vi "CSM - Request CSM to Post Message.vi"(4 "Immediately?(F)":bool, 6 "Without Reply?(F)":bool, 7 "Module Name":string, 8 "Error In (no error)":errorcluster, 9 "Target Module(\"\" by Default)":string, 10 "Arguments (\"\")":string, 11 "State":string) -> (0 "error out":errorcluster)   [LabVIEW 2020, in "Communicable State Machine.lvlib"]
doc: "Request CSM to Post a message to CSM specified. This is usually used in sub-loops with a CSM for acting as a holistic module.\n\n<b>Inputs:</b>\n - <b>Status</b>: Message to post.\n - <b>Arguments (\"\")</b>: Argument of the message.\n - <b>Target Module</b>:Target CSM module name.\n - <b>Module Name</b>:Host Module Name\n - <b>Error In (no error)</b>: Error cluster\n\n<b>Outputs:</b>\n - <b>error out</b>: Error cluster"
uses:
  Communicable State Machine.lvlib
  _CSM_MSG_TYPE.ctl
  CSM - Message Type.ctl
  _Cross CSM State Data.ctl
  _Cross CSM State Response.ctl
  _CSM_Response Source Message.ctl
  _CSMOFGVOPER.ctl
  Priority Queue.lvclass/Priority Queue.ctl
  Priority Queue.lvclass
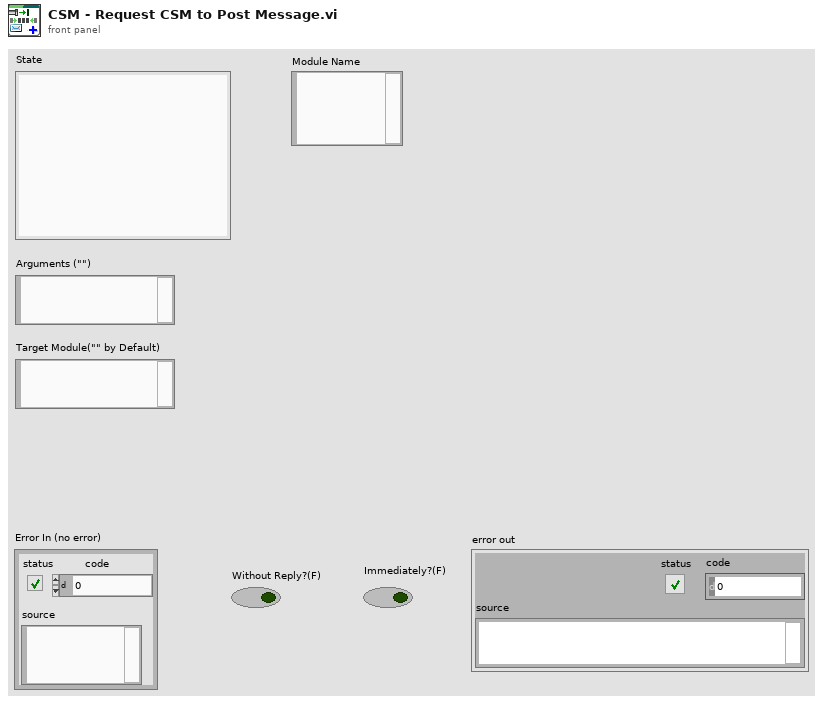
[diagram p1: front panel]
types:
  T1 = typedef "Communicable State Machine.lvlib/_CSM_MSG_TYPE.ctl" = enum16{"Sync Message(-@)", "Async Message(->)", "Async without Response(->|)", "Async Response", "Broadcast(-><all>)", "Broadcast(-><status>)", "Broadcast(-><interrupt>)", "Append to JKISM States", "Append to JKISM States(High Priority)"}
  T2 = typedef "Communicable State Machine.lvlib/CSM - Message Type.ctl" = enum16{"Async", "Async without Reply", "Sync"}
  T3 = typedef "Communicable State Machine.lvlib/_Cross CSM State Data.ctl" = cluster{"Msg Type":T1, "state":string, "args":string, "source":string, "RespQ":refnum<queue>, "Response For Message":T4, "Target":string}
  T4 = typedef "Communicable State Machine.lvlib/_CSM_Response Source Message.ctl" = cluster{"‘State":string, "’Arguments":string, "’Error":errorcluster}
  T5 = typedef "Communicable State Machine.lvlib/_CSMOFGVOPER.ctl" = enum16{"Create If not Exist", "Get By Name", "List", "Check If Name Exists", "Release", "Module Status", "Create Status Event Handler", "Destroy Status Event Handler"}
  T6 = typedef "Communicable State Machine.lvlib/_CSMObj.ctl" = cluster{"Requested Name":string, "Module Name":string, "Mode":T7, "Queue":refnum<class "Priority Queue.lvclass">, "CSM-Data":refnum<data-value>, "User Event":refnum<user-event>, "Status Change Event":refnum<user-event>, "Allowed Messages":string[], "Mode-Data":refnum<data-value>, "Group Name":string, "Exit Event":refnum<user-event>}
  T7 = typedef "Communicable State Machine.lvlib/_CSM_MODE.ctl" = enum16{"Not Exist", "Stand Alone", "CSM", "Worker Agent", "Worker", "Chain", "Chain Node"}
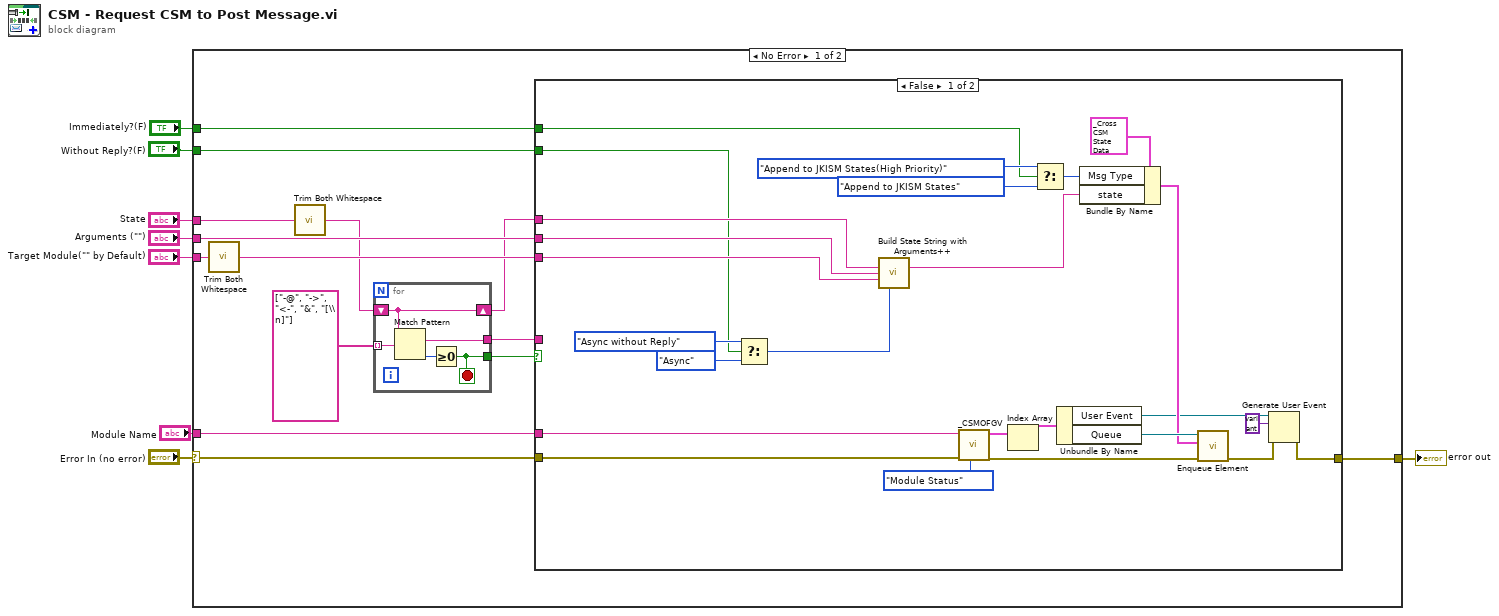
[diagram p0: block diagram]
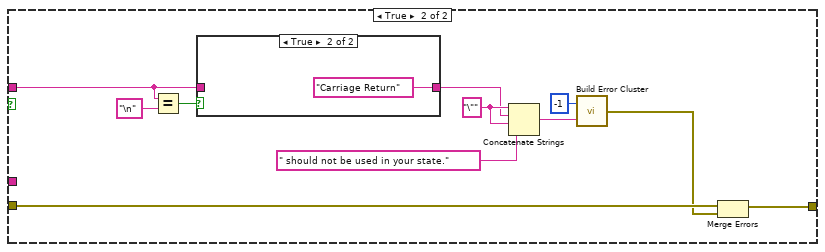
[diagram p2: hidden frame]
diagram:
  n1 = case shown="No Error" "Error In (no error)" {
    selector: "Error In (no error)" -> [w20 w66]
    tunnel: "State" -> [w17 _]
    tunnel: [w21 w66] -> w6
    tunnel: "Arguments (\"\")" -> [w18 _]
    tunnel: "Target Module(\"\" by Default)" -> [w22 _]
    tunnel: "Module Name" -> [w16 _]
    tunnel: "Without Reply?(F)" -> [w15 _]
    tunnel: "Immediately?(F)" -> [w9 _]
    frame No Error {
      n2 = call "Trim Both Whitespace.vi"("string"=w22) -> ("trimmed string"=w19:string)  [unwired: 1 in]
      n3 = call "Trim Both Whitespace.vi"("string"=w17) -> ("trimmed string"=w10:string)  [unwired: 1 in]
      n4 = for {
        shift-right: [w65] -> w13
        shift-left: w10 -> [w65]
        tunnel: string[] ["-@", "->", "<-", "&", "[\\n]"] -> [w64] mode=indexing
        tunnel: [w62] -> w11
        tunnel: [w61] -> w12
        stop <- w61 stop-if-true
        n5 = Match Pattern(string=w65, regular expression=w64) -> (match substring=w62:string, offset past match=w63:i32)  [unwired: 1 in, 2 out]
        n6 = Greater Or Equal To 0?(x=w63) -> (x >= 0?=w61:bool)
      }
      n7 = case shown="False" w12 {
        tunnel: w18 -> [w32 _]
        tunnel: w19 -> [w31 _]
        tunnel: [w36 w50] -> w21
        tunnel: w20 -> [w40 w51]
        tunnel: w13 -> [w33 _]
        tunnel: w11 -> [_ w48]
        tunnel: w16 -> [w38 _]
        tunnel: w15 -> [w24 _]
        tunnel: w9 -> [w25 _]
        frame False {
          n8 = Select(t=CSM_-_Message_Type."Async without Reply" ("Type"), s=w24, f=CSM_-_Message_Type."Async" ("Type")) -> (s? t:f=w23:T2)
          n9 = call "Build State String with Arguments++.vi"("State"=w33, "Arguments (\"\")"=w32, "Target Module (\"\")"=w31, "Type"=w23) -> ("State with Arguments"=w30:string)  [unwired: 11 in]
          n10 = call "_CSMOFGV.vi"("Operation"=_CSMOFGVOPER."Module Status", "Error in"=w40, "Name(\"\" to use uuid) in"=w38) -> ("Error out"=w41:errorcluster, "Array"=w46:T6[])  [unwired: 6 in, 1 out]
          n11 = Index Array(array=w46) -> (element=w45:T6)  [unwired: 1 in]
          n12 = Select(t=_CSM_MSG_TYPE."Append to JKISM States(High Priority)" ("Msg Type"), s=w25, f=_CSM_MSG_TYPE."Append to JKISM States" ("Msg Type")) -> (s? t:f=w37:T1)
          n13 = Unbundle By Name(w45) -> ("User Event"=w35:refnum<user-event>, "Queue"=w44:refnum<class "Priority Queue.lvclass">)
          n14 = Bundle By Name(cluster=T3 {"Msg Type"=enum."Sync Message(-@)", "state"="", "args"="", "source"="", "RespQ"=refnum, "Response For Message"={"‘State"="", "’Arguments"="", "’Error"={"status"=FALSE, "code"=0, "source"=""}}, "Target"=""} ("element"), "Msg Type"=w37, "state"=w30) -> (w42:T3)
          n15 = call "Enqueue Element.vi"("error in (no error)"=w41, "Cross JKI State Machine State"=w42, "Priority Queue"=w44) -> ("error out"=w39:errorcluster)  [unwired: 7 in, 1 out]
          n16 = Generate User Event(user event=w35, event data cluster=variant ("event data"), error in=w39) -> (error out=w36:errorcluster)  [unwired: 1 in, 1 out]
        }
        frame True {
          w55 = "\"" ("string")
          n17 = Equal?(x=w48, y="\n" ("regular expression")) -> (x = y?=w52:bool)
          n18 = case shown="True" w52 {
            tunnel: [w59 "Carriage Return" ("State")] -> w54
            tunnel: w48 -> [w59 _]
            frame False {
            }
            frame True {
            }
          }
          n19 = Concatenate Strings(w55, w54, w55, " should not be used in your state." ("String to Prepend to source (\"\")")) -> (w56:string)
          n20 = call "Build Error Cluster.vi"("String to Prepend to source (\"\")"=w56, "code"=-1) -> ("error out"=w49:errorcluster)
          n21 = Merge Errors(w51, w49) -> (w50:errorcluster)
        }
      }
    }
    frame Error {
    }
  }
  "error out" <- w6
